vi "Initialize.vi"(8 "error in (no error)":errorcluster, 11 "Error Handler in":refnum<class "Error Handler.lvclass">) -> (0 "error out":errorcluster, 3 "Error Handler out":refnum<class "Error Handler.lvclass">)   [LabVIEW 2021, in "Error Handler.lvlib" / "Error Handler.lvclass"]
uses:
  Error Handler.lvclass
  Error Handler.lvclass/Error Handler.ctl
  public types/response.ctl
  Error Handler.lvlib
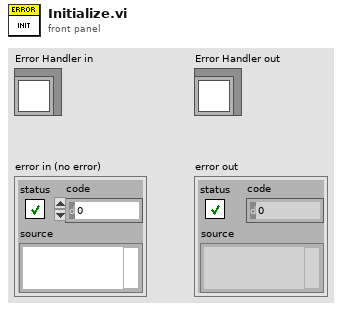
[diagram p1: front panel]
types:
  T1 = typedef "Error Handler.lvlib/response.ctl" = enum16{"log", "log & popup", "log & exit", "log & popup & exit", "popup", "popup & exit", "exit", "ignore"}
  T2 = cluster{"status":bool, "code":i32, "source":string, "timestamp":i32}
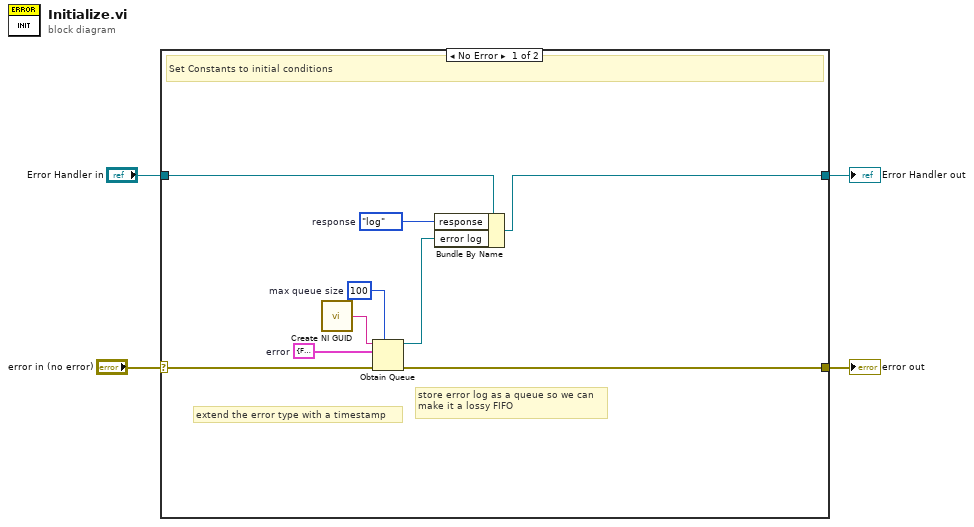
[diagram p0: block diagram]
diagram:
  n1 = case shown="No Error" "error in (no error)" {
    selector: "error in (no error)" -> [w13 w15]
    tunnel: [w12 w15] -> w3
    tunnel: [w7 w14] -> w1
    tunnel: "Error Handler in" -> [w9 w14]
    frame No Error {
      w5 = response."log"  # response
      w10 = 100  # max queue size
      w11 = T2 {"status"=FALSE, "code"=0, "source"="", "timestamp"=0}  # error
      # "store error log as a queue so we can\nmake it a lossy FIFO"
      # "extend the error type with a timestamp"
      # "Set Constants to initial conditions"
      n2 = call <vilib>:"Create NI GUID.vi"() -> ("NI GUID"=w8:string)
      n3 = Obtain Queue(max queue size (-1, unlimited)=w10, name (unnamed)=w8, element data type=w11, error in (no error)=w13) -> (queue out=w6:refnum<queue>, error out=w12:errorcluster)  [unwired: 1 in, 1 out]
      n4 = Bundle By Name(cluster=w9, "response"=w5, "error log"=w6) -> (w7:refnum<class "Error Handler.lvclass">)
    }
    frame Error {
    }
  }
  "error out" <- w3
  "Error Handler out" <- w1
